vi "DetectingVailableWork.vi"(9 "inputCondition":T1, 10 "Reset":bool) -> (2 "Progressing":bool)   [LabVIEW 2024]
uses:
  Control/DetectingVailableWorkState.ctl
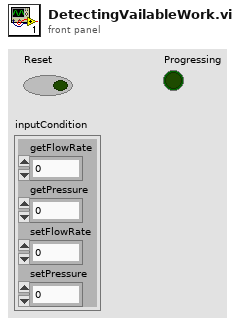
[diagram p1: front panel]
types:
  T1 = cluster{"getFlowRate":dbl, "getPressure":dbl, "setFlowRate":dbl, "setPressure":dbl}
  T2 = typedef "DetectingVailableWorkState.ctl" = enum16{"Ready", "Detecting FlowRate", "Detecing Pressure"}
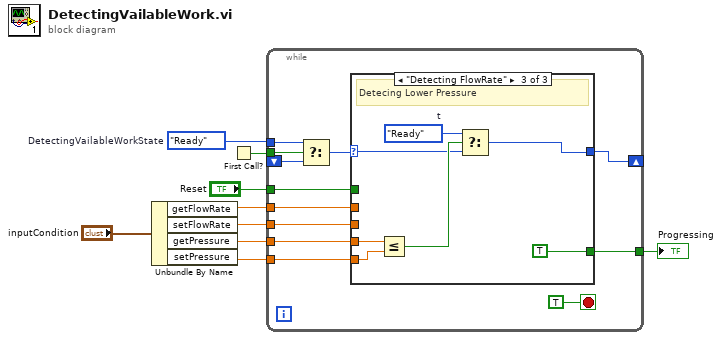
[diagram p0: block diagram]
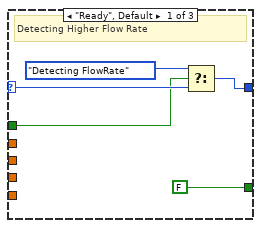
[diagram p2: hidden frame]
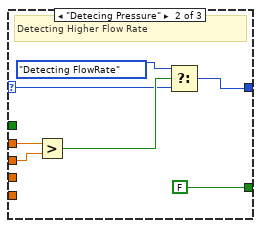
[diagram p3: hidden frame]
diagram:
  w2 = DetectingVailableWorkState."Ready"  # DetectingVailableWorkState
  n1 = Unbundle By Name("inputCondition") -> ("getFlowRate"=w6:dbl, "setFlowRate"=w5:dbl, "getPressure"=w4:dbl, "setPressure"=w3:dbl)
  n2 = First Call?() -> (First Call?: T/F=w9:bool)
  n3 = while {
    shift-right: [w16] -> _
    shift-left: _ -> [w18]
    tunnel: w9 -> [w20]
    tunnel: w2 -> [w19]
    tunnel: w6 -> [w15]
    tunnel: w4 -> [w14]
    tunnel: w5 -> [w12]
    tunnel: w3 -> [w13]
    tunnel: [w11] -> w8
    tunnel: "Reset" -> [w10]
    stop <- TRUE stop-if-true
    n4 = Select(t=w19, s=w20, f=w18) -> (s? t:f=w17:T2)
    n5 = case shown="\"Detecting FlowRate\"" w17 {
      selector: w17 -> [w26 w30 w36]
      tunnel: [w25 w29 w35] -> w16
      tunnel: w15 -> [_ w33 _]
      tunnel: w14 -> [_ _ w40]
      tunnel: w13 -> [_ _ w39]
      tunnel: w12 -> [_ w32 _]
      tunnel: [FALSE FALSE TRUE] -> w11
      tunnel: w10 -> [w22 _ _]
      frame "Ready", Default {
        # "Detecting Higher Flow Rate"
        n6 = Select(t=DetectingVailableWorkState."Detecting FlowRate" ("DetectingVailableWorkState"), s=w22, f=w26) -> (s? t:f=w25:T2)
      }
      frame "Detecing Pressure" {
        # "Detecting Higher Flow Rate"
        n7 = Greater?(x=w33, y=w32) -> (0:w31:bool)
        n8 = Select(t=DetectingVailableWorkState."Detecting FlowRate" ("DetectingVailableWorkState"), s=w31, f=w30) -> (s? t:f=w29:T2)
      }
      frame "Detecting FlowRate" {
        w34 = DetectingVailableWorkState."Ready"  # t
        # "Detecing Lower Pressure"
        n9 = Less Or Equal?(x=w40, y=w39) -> (x <= y?=w37:bool)
        n10 = Select(t=w34, s=w37, f=w36) -> (s? t:f=w35:T2)
      }
    }
  }
  "Progressing" <- w8
